vi "Expt 12.vi"() -> ()   [LabVIEW 2020]
uses:
  <vilib>/Utility/file.llb/Write Delimited Spreadsheet (string).vi
panel:
  out "current time":timestamp
  in  "file path (dialog if empty)":path
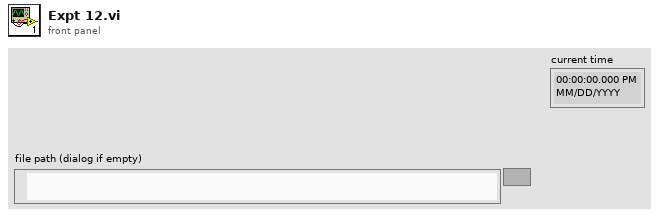
[diagram p1: front panel]
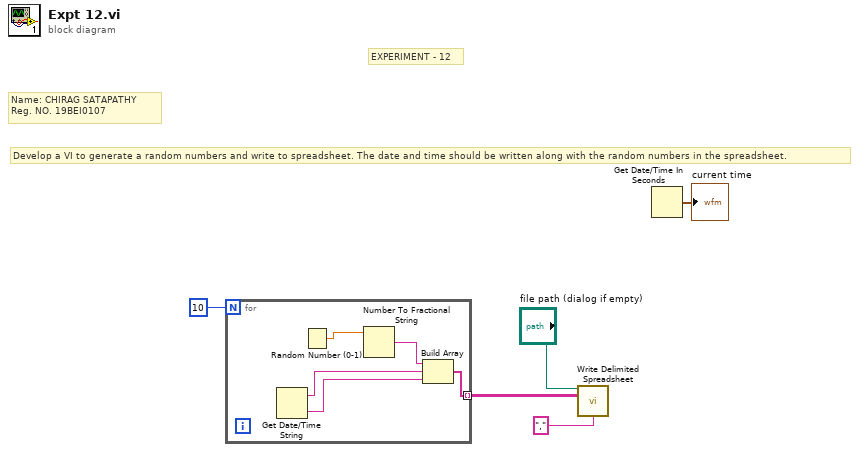
[diagram p0: block diagram]
diagram:
  # "Develop a VI to generate a random numbers and write to spreadsheet. The date and time should be written along with the random numbers in the spreadsheet."
  # "Name: CHIRAG SATAPATHY\nReg. NO. 19BEI0107"
  # "EXPERIMENT - 12"
  n1 = for {
    N: 10 -> [_]
    tunnel: [w7] -> w1 mode=indexing
    n2 = Get Date/Time String() -> (date string=w9:string, time string=w8:string)  [unwired: 3 in]
    n3 = Random Number (0-1)() -> (number: 0 to 1=w6:dbl)
    n4 = Number To Fractional String(number=w6) -> (F-format string=w10:string)  [unwired: 3 in]
    n5 = Build Array(w10, w9, w8) -> (w7:string[])
  }
  n6 = call-poly <vilib>:"Write Delimited Spreadsheet.vi"("file path (dialog if empty)"="file path (dialog if empty)", "2D data"=w1, "delimiter (\\t)"="," ("delimiter (\\t)")) -> ()  [unwired: 11 in, 2 out]
  n7 = Get Date/Time In Seconds() -> (seconds since 1Jan1904=→"current time":timestamp)
